vi "create face names.vi"(8 "error out 2":errorcluster, 11 "Scene:New Object 2":refnum<vi>) -> (0 "error out":errorcluster, 3 "Scene:New Object":refnum<vi>)   [LabVIEW 2019]
uses:
  <vilib>/picture/3D Picture Control/Object/Create Object (name).vi
  <vilib>/picture/3D Picture Control/NI_3D Picture Control.lvlib
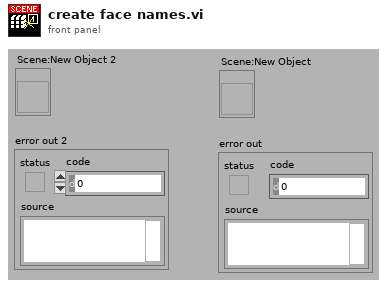
[diagram p1: front panel]
types:
  T1 = cluster{"Axis":cluster{"X":sgl, "Y":sgl, "Z":sgl}, "Angle":sgl}[]
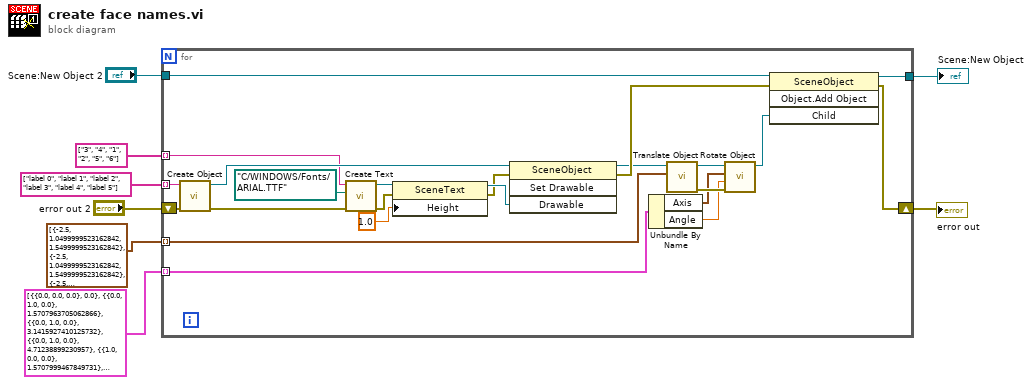
[diagram p0: block diagram]
diagram:
  n1 = for {
    tunnel: "Scene:New Object 2" -> [w30]
    shift-right: [w19] -> w8
    shift-left: "error out 2" -> [w31]
    tunnel: string[] ["label 0", "label 1", "label 2", "label 3", "label 4", "label 5"] -> [w28] mode=indexing
    tunnel: T1 [{"Axis"={"X"=0.0, "Y"=0.0, "Z"=0.0}, "Angle"=0.0}, {"Axis"={"X"=0.0, "Y"=1.0, "Z"=0.0}, "Angle"=1.5707964}, {"Axis"={"X"=0.0, "Y"=1.0, "Z"=0.0}, "Angle"=3.1415927}, {"Axis"={"X"=0.0, "Y"=1.0, "Z"=0.0}, "Angle"=4.712389}, {"Axis"={"X"=1.0, "Y"=0.0, "Z"=0.0}, "Angle"=1.5708}, {"Axis"={"X"=1.0, "Y"=0.0, "Z"=0.0}, "Angle"=4.71239}] -> [w24] mode=indexing
    tunnel: cluster{"X":sgl, "Y":sgl, "Z":sgl}[] [{"X"=-2.5, "Y"=1.05, "Z"=1.55}, {"X"=-2.5, "Y"=1.05, "Z"=1.55}, {"X"=-2.5, "Y"=1.05, "Z"=1.55}, {"X"=-2.5, "Y"=1.05, "Z"=1.55}, {"X"=2.5, "Y"=1.05, "Z"=-1.55}, {"X"=-2.5, "Y"=1.05, "Z"=-1.55}] -> [w22] mode=indexing
    tunnel: [w20] -> w4
    tunnel: string[] ["3", "4", "1", "2", "5", "6"] -> [w17] mode=indexing
    n2 = call-poly <vilib>:"Create Object.vi"("error in (no error)"=w31, "Name"=w28) -> ("error out"=w12:errorcluster, "Scene:New Object"=w18:refnum<vi>)  [unwired: 8 in]
    n3 = call <vilib>:"Create Text.vi"("error in (no error)"=w12, "Path to font file"=path "C:/WINDOWS/Fonts/ARIAL.TTF", "Text"=w17) -> ("error out"=w11:errorcluster, "New Text Refnum"=w16:refnum<vi>)  [unwired: 7 in]
    n4 = property class="SceneText"(reference=w16, error in=w11, "Height"=sgl 1.0 ("Character Size")) -> (reference out=w15:refnum<vi>, error out=w10:errorcluster)
    n5 = invoke class="SceneObject" method="Set Drawable"(reference=w18, error in=w10, "Drawable"=w15) -> (reference out=w27:refnum<vi>, error out=w29:errorcluster)  [unwired: 1 in, 2 out]
    n6 = Unbundle By Name(w24) -> ("Axis"=w23:cluster{"X":sgl, "Y":sgl, "Z":sgl}, "Angle"=w21:sgl)
    n7 = call <vilib>:"Translate Object.vi"("Translation"=w22, "Scene.Object In"=w27) -> ("error out"=w25:errorcluster, "Scene.Object Out"=w26:refnum<vi>)  [unwired: 8 in]
    n8 = call <vilib>:"Rotate Object.vi"("error in (no error)"=w25, "Angle"=w21, "Axis"=w23, "Scene.Object In"=w26) -> ("Scene.Object Out"=w13:refnum<vi>)  [unwired: 6 in, 1 out]
    n9 = invoke class="SceneObject" method="Object.Add Object"(reference=w30, error in=w29, "Child"=w13) -> (reference out=w20:refnum<vi>, error out=w19:errorcluster)  [unwired: 1 in, 2 out]
  }
  "error out" <- w8
  "Scene:New Object" <- w4
